vi "Set Build Specification Version (path).vi"(6 "Build Specification Version":T1, 8 "error in (no error)":errorcluster, 9 "Name of target (My Computer)":string="My Computer", 10 "Name of build specification":string, 11 "Path to project":path) -> (0 "error out":errorcluster)   [LabVIEW 2020, in "NI_App_Builder_API.lvlib"]
doc: "Sets the version information of a build specification. This VI sets the <B>Major, Minor, Fix</B>, and <B>Build</B> version numbers, which correspond to the version numbers on the <B>Version Information</B> page of the properties dialog box for the build specification. LabVIEW saves version information automatically only if you wire a path to this VI. Therefore, if you wire a project reference to this VI, you must manually save the project after you set the version information."
uses:
  <vilib>/AppBuilder/AB_API_Simple/NI_App_Builder_API.lvlib
  <vilib>/AppBuilder/AB_API_Simple/Build Specification Version.ctl
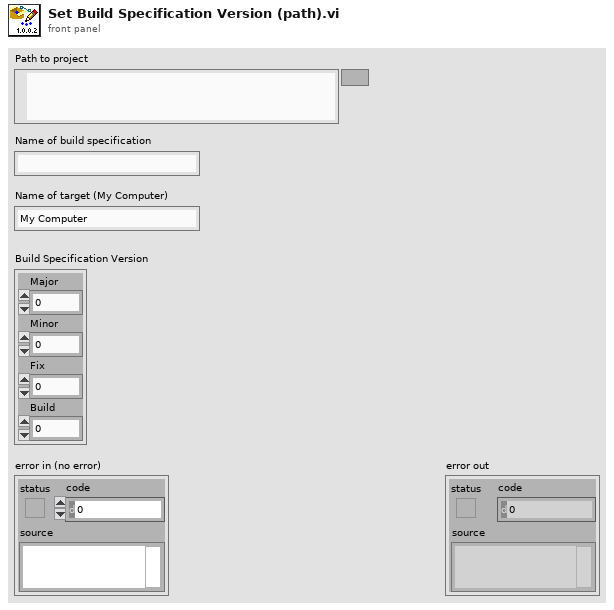
[diagram p1: front panel]
types:
  T1 = typedef "NI_App_Builder_API.lvlib/Build Specification Version.ctl" = cluster{"Major":u16, "Minor":u16, "Fix":u16, "Build":u16}
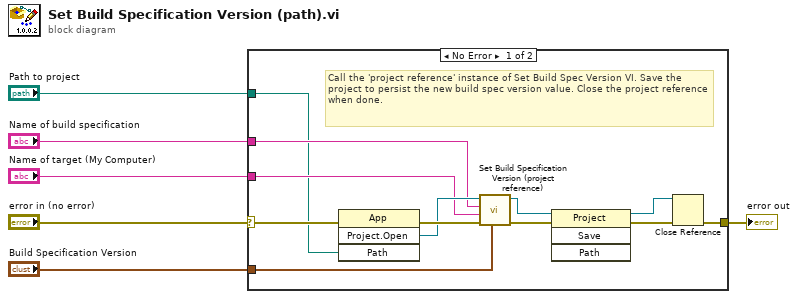
[diagram p0: block diagram]
diagram:
  n1 = case shown="No Error" "error in (no error)" {
    selector: "error in (no error)" -> [w18 w19]
    tunnel: "Path to project" -> [w11 _]
    tunnel: "Name of target (My Computer)" -> [w12 _]
    tunnel: "Name of build specification" -> [w13 _]
    tunnel: [w14 w19] -> w1
    tunnel: "Build Specification Version" -> [w10 _]
    frame No Error {
      # "Call the 'project reference' instance of Set Build Spec Version VI. Save the project to persist the new build spec version value. Close the project reference when done."
      n2 = invoke class="App" method="Project.Open"(error in=w18, "Path"=w11) -> (error out=w17:errorcluster, "Project:Open"=w16:refnum<vi>)  [unwired: 2 in, 2 out]
      n3 = call <vilib>:"Set Build Specification Version (project reference).vi"("Build Specification Version"=w10, "error in"=w17, "Name of target (My Computer)"=w12, "Name of build specification"=w13, "Project reference"=w16) -> ("error out"=w15:errorcluster, "dup Project reference"=w8:refnum<vi>)  [unwired: 5 in]
      n4 = invoke class="Project" method="Save"(reference=w8, error in=w15) -> (reference out=w7:refnum<vi>, error out=w9:errorcluster)  [unwired: 2 in, 2 out]
      n5 = Close Reference(reference=w7, error in (no error)=w9) -> (error out=w14:errorcluster)
    }
    frame Error {
    }
  }
  "error out" <- w1
